vi "Last Notification.vi"(8 "error in (no error)":errorcluster, 11 "NotifierMessenger in":refnum<class "NotifierMessenger.lvclass">) -> (0 "error out":errorcluster, 2 "Message":refnum<class "MSG.lvclass">, 3 "NotifierMessenger out":refnum<class "NotifierMessenger.lvclass">)   [LabVIEW 2011, in "Messenging.lvlib" / "NotifierMessenger.lvclass"]
uses:
  NotifierMessenger.lvclass
  TextVarientMessage/MSG.lvclass
  NotifierMessenger.lvclass/NotifierMessenger.ctl
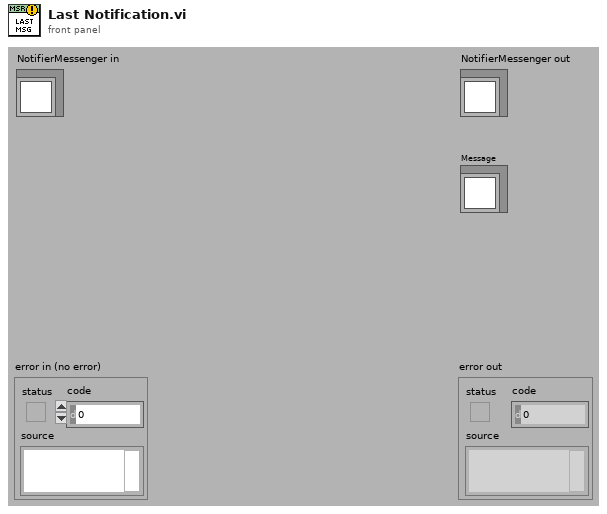
[diagram p1: front panel]
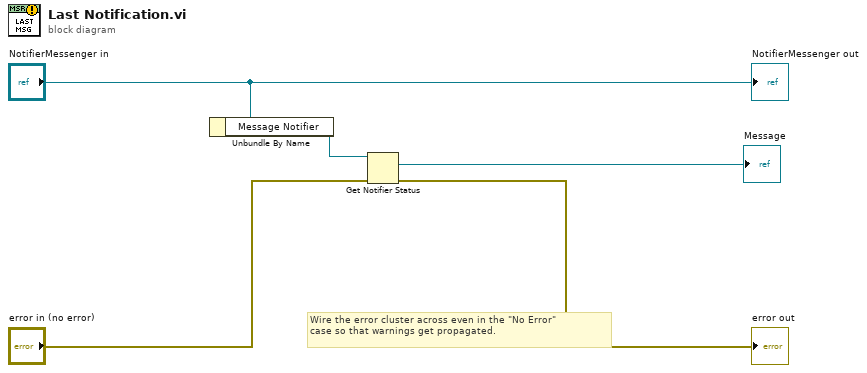
[diagram p0: block diagram]
diagram:
  # "Wire the error cluster across even in the \"No Error\"\ncase so that warnings get propagated."
  n1 = Unbundle By Name("NotifierMessenger in") -> ("Message Notifier"=w1:refnum<notifier>)
  n2 = Get Notifier Status(notifier=w1, error in (no error)="error in (no error)") -> (current notification=→"Message":refnum<class "MSG.lvclass">, error out=→"error out":errorcluster)  [unwired: 3 out]
  "NotifierMessenger out" <- "NotifierMessenger in"
